vi "TestCaseTimer.vi"() -> ()   [LabVIEW 2026]
panel:
  out "Test State Timer":dbl format="%#_3f"
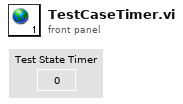
[diagram p1: front panel]
diagram:
